vi "iBisquare Weights.vi"(8 "my eps":dbl, 11 "Array":dbl[](array[numeric])) -> (3 "Weights":dbl[](array[numeric]))   [LabVIEW 2020]
uses:
  <vilib>/Analysis/NI_AALBase.lvlib
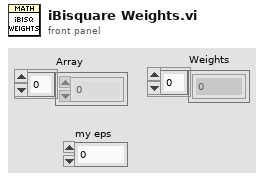
[diagram p1: front panel]
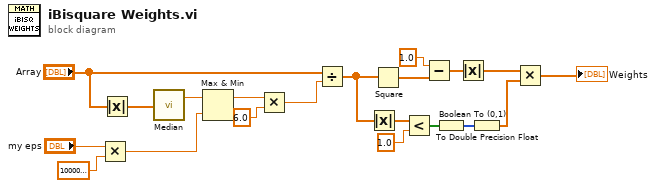
[diagram p0: block diagram]
diagram:
  n1 = Multiply(x="my eps", y=100000000.0) -> (x*y=w16:dbl)
  n2 = Absolute Value(x="Array") -> (abs(x)=w18:dbl[])
  n3 = call <vilib>:"Median.vi"("X"=w18) -> ("median"=w17:dbl)  [unwired: 1 out]
  n4 = Max & Min(x=w17, y=w16) -> (max(x,y)=w15:dbl)  [unwired: 1 out]
  n5 = Multiply(x=w15, y=6.0) -> (x*y=w12:dbl)
  n6 = Divide(x="Array", y=w12) -> (x/y=w8:dbl[])
  n7 = Absolute Value(x=w8) -> (abs(x)=w7:dbl[])
  n8 = Square(x=w8) -> (x^2=w10:dbl[])
  n9 = Less?(x=w7, y=1.0) -> (x < y?=w5:bool[])
  n10 = Subtract(x=1.0, y=w10) -> (x-y=w9:dbl[])
  n11 = Boolean To (0,1)(Boolean=w5) -> (0, 1=w4:i16[])
  n12 = Absolute Value(x=w9) -> (abs(x)=w3:dbl[])
  n13 = To Double Precision Float(number=w4) -> (double precision float=w2:dbl[])
  n14 = Multiply(x=w3, y=w2) -> (x*y=→"Weights":dbl[])
